vi "ADAMPacer.vi"(4 "Scan Period":dbl format="%.2f", 5 "Previous Scan Value":dbl format="%.2f", 6 "Present scan array":dbl[](array[numeric]) format="%.2f", 7 "Value to Output":dbl format="%.2f", 8 "Ch Description":T1={"Ch Name"="", "Type"="", "Function"=enum."Analogue Input", "Ch State"=enum."On", "Calibration type"="", "A"=0.0, "B"=0.0, "C"=0.0, "D"=0.0, "Comments"="", "Address"={"Main"=0, "Ch."=0, "Sub"=0, "Port Name"=""}, "String"="", "Duty"=65535} {"Duty" format="%016b"; "D" format="%#_5g"; "C" format="%#_5g"; "B" format="%#_5g"; "A" format="%#_5g"}, 9 "Ch names":string[](array[string])) -> (0 "Scan comment":string, 1 "slug(s)":dbl format="%.3f", 3 "HelpText":string)   [LabVIEW 2021]
uses:
  ADAM Client/Sub VIs/ADAM Controls/Ch_description_ADAM.ctl
  ADAM Client/Sub VIs/ADAM Controls/Module_type_ADAM.ctl
  ADAM Client/Sub VIs/ADAM Controls/Function_ADAM.ctl
  ADAM Client/Sub VIs/ADAM Controls/Channel_State.ctl
  ADAM Client/Sub VIs/ADAM Controls/Calib_type_ADAM.ctl
  ADAM Client/Sub VIs/ADAM Controls/Address.ctl
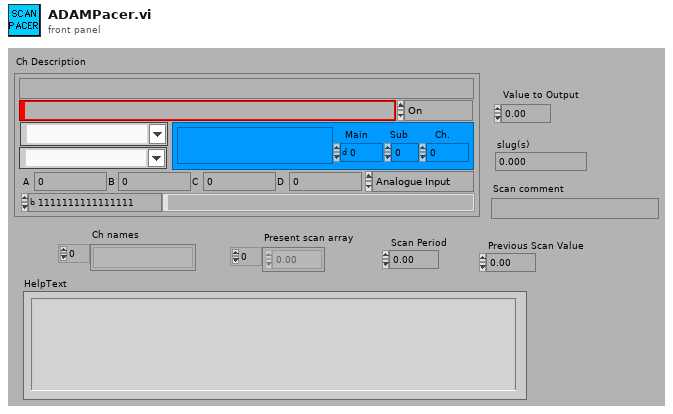
[diagram p1: front panel]
types:
  T1 = typedef "Ch_description_ADAM.ctl" = cluster{"Ch Name":string, "Type":T2, "Function":T3, "Ch State":T4, "Calibration type":T5, "A":dbl, "B":dbl, "C":dbl, "D":dbl, "Comments":string, "Address":T6, "String":string, "Duty":u16}
  T2 = typedef "Module_type_ADAM.ctl" = string
  T3 = typedef "Function_ADAM.ctl" = enum16{"Analogue Input", "Digital Input", "Event counter", "Event rate", "Analogue Output", "Digital Output", "Relay Output"}
  T4 = typedef "Channel_State.ctl" = enum16{"On", "Off", "Always On", "Always Off"}
  T5 = typedef "Calib_type_ADAM.ctl" = string
  T6 = typedef "Address.ctl" = cluster{"Main":i32, "Ch.":i32, "Sub":i32, "Port Name":string}
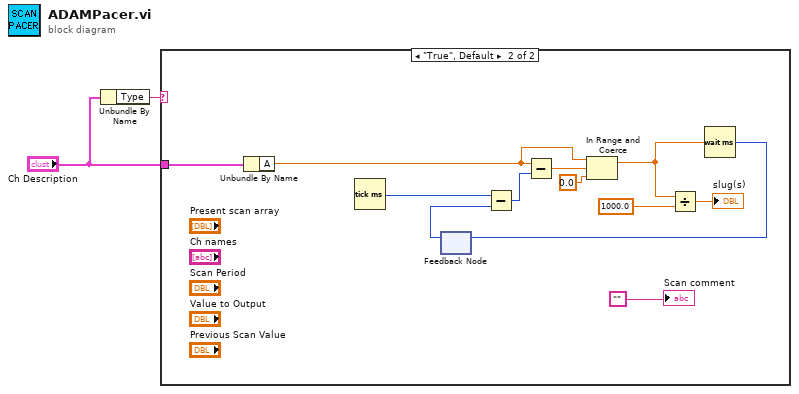
[diagram p0: block diagram]
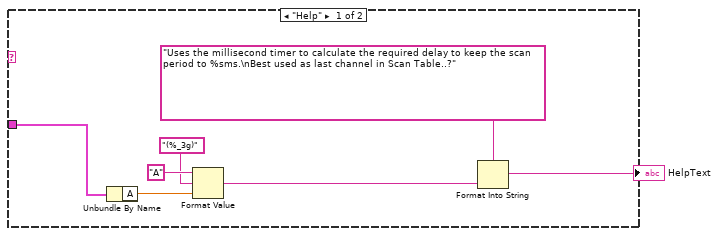
[diagram p2: hidden frame]
diagram:
  n1 = Unbundle By Name("Ch Description") -> ("Type"=w2:T2)
  n2 = case shown="\"True\", Default" w2 {
    tunnel: "Ch Description" -> [w6 w15]
    frame "Help" {
      n3 = Unbundle By Name(w6) -> ("A"=w8:dbl)
      n4 = Format Value(string ("")="A", format string="(%_3g)", value (0)=w8) -> (output string=w4:string)
      n5 = Format Into String(format string="Uses the millisecond timer to calculate the required delay to keep the scan period to %sms.\nBest used as last channel in Scan Table..?", w4) -> (resulting string=→"HelpText":string)  [unwired: 2 in, 1 out]
    }
    frame "True", Default {
      n6 = Unbundle By Name(w15) -> ("A"=w17:dbl)
      n7 = Tick Count (ms)() -> (millisecond timer value=w13:u32)
      n8 = feedback #1() -> (w14:u32)  [unwired: 1 in]
      n9 = Subtract(x=w13, y=w14) -> (x-y=w20:u32)
      n10 = Subtract(x=w17, y=w20) -> (x-y=w19:dbl)
      n11 = In Range and Coerce(upper limit=w17, x=w19, lower limit=0.0) -> (coerced(x)=w16:dbl)  [unwired: 1 out]
      n12 = Divide(x=w16, y=1000.0) -> (x/y=→"slug(s)":dbl)
      n13 = Wait (ms)(milliseconds to wait=w16) -> (millisecond timer value=w12:u32)
      n14 = feedback-in #1(w12) -> ()
      "Scan comment" <- ""
    }
  }
